vi "Set Destination Directory.vi"(7 "Destination Type":string="LLB", 8 "error in (no error)":errorcluster, 10 "Directory Path":path, 11 "BuildSpec in":refnum<vi>) -> (0 "error out":errorcluster, 3 "BuildSpec out":refnum<vi>)   [LabVIEW 2019, in "Project Sync Tools.lvclass"]
uses:
  Project Sync Tools.lvclass
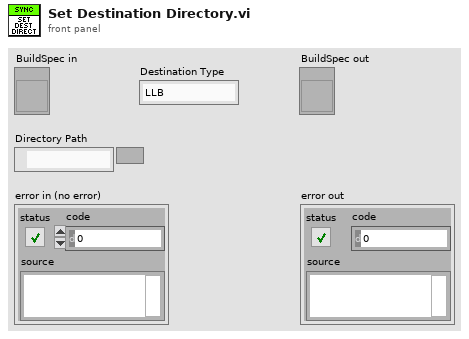
[diagram p1: front panel]
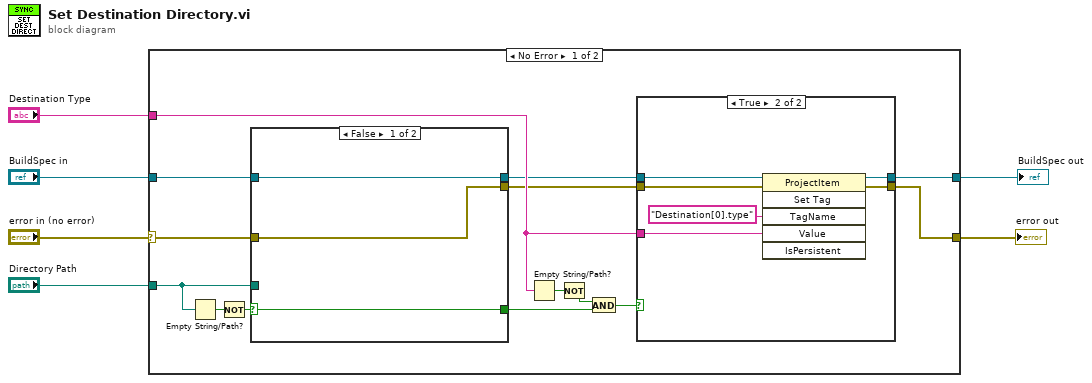
[diagram p0: block diagram]
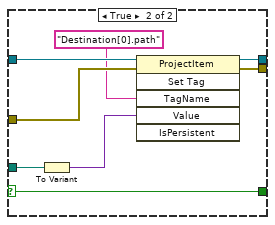
[diagram p3: hidden frame]
diagram:
  n1 = case shown="No Error" "error in (no error)" {
    selector: "error in (no error)" -> [w17 w40]
    tunnel: [w20 w40] -> w6
    tunnel: [w19 w41] -> w5
    tunnel: "BuildSpec in" -> [w18 w41]
    tunnel: "Directory Path" -> [w16 _]
    tunnel: "Destination Type" -> [w15 _]
    frame No Error {
      n2 = Empty String/Path?(string/path=w16) -> (empty?=w14:bool)
      n3 = Not(x=w14) -> (.not. x?=w10:bool)
      n4 = case shown="False" w10 {
        selector: w10 -> [w29 w32]
        tunnel: w18 -> [w31 w39]
        tunnel: w17 -> [w30 w38]
        tunnel: w16 -> [_ w37]
        tunnel: [w30 w36] -> w12
        tunnel: [w31 w33] -> w11
        tunnel: [w29 w32] -> w7
        frame False {
        }
        frame True {
          n5 = To Variant(anything=w37) -> (Variant=w34:variant)
          n6 = invoke class="ProjectItem" method="Set Tag"(reference=w39, error in=w38, "TagName"="Destination[0].path" ("Tag Name"), "Value"=w34) -> (reference out=w33:refnum<vi>, error out=w36:errorcluster)  [unwired: 2 in, 4 out]
        }
      }
      n7 = Empty String/Path?(string/path=w15) -> (empty?=w13:bool)
      n8 = Not(x=w13) -> (.not. x?=w9:bool)
      n9 = And(x=w9, y=w7) -> (x .and. y?=w8:bool)
      n10 = case shown="True" w8 {
        tunnel: [w21 w28] -> w20
        tunnel: [w22 w27] -> w19
        tunnel: w15 -> [_ w26]
        tunnel: w12 -> [w21 w25]
        tunnel: w11 -> [w22 w24]
        frame False {
        }
        frame True {
          n11 = invoke class="ProjectItem" method="Set Tag"(reference=w24, error in=w25, "TagName"="Destination[0].type" ("Tag Name"), "Value"=w26) -> (reference out=w27:refnum<vi>, error out=w28:errorcluster)  [unwired: 2 in, 4 out]
        }
      }
    }
    frame Error {
    }
  }
  "error out" <- w6
  "BuildSpec out" <- w5
